vi "Add Transfer Group.vi"(8 "error in (no error)":errorcluster, 9 "Transfer Group":refnum<class "Transfer Group.lvclass">, 10 "parent tag":string, 11 "TreeControl in":refnum<vi>) -> (0 "error out":errorcluster, 2 "new item tag":string, 3 "TreeControl out":refnum<vi>)   [LabVIEW 2021, in "DSF Core.lvlib"]
uses:
  DSF Core.lvlib
  Classes/Transfer Group/Transfer Group.lvclass
  ID to Tree Items/Tree Item Type.ctl
  Classes/Transfer Group/Transfer Group.lvclass/Transfer Group.ctl
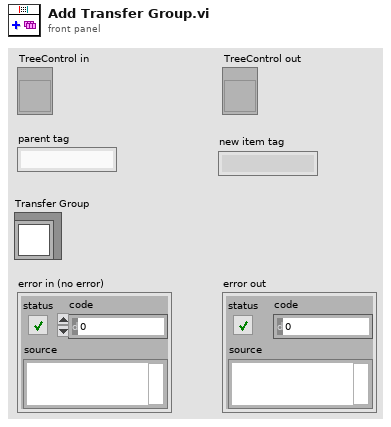
[diagram p1: front panel]
types:
  T1 = typedef "DSF Core.lvlib/Tree Item Type.ctl" = enum16{"Framework", "Plugin Group", "Plugin", "Group", "Transfer", "Buffer", "Channel"}
  T2 = typedef "DSF Core.lvlib/Tree Item.ctl" = cluster{"Left Cell String":string, "Child Text":string[], "Child Tag":string, "Glyph Index":i32}
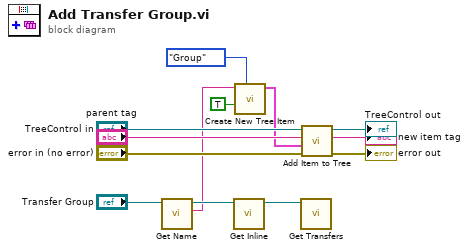
[diagram p0: block diagram]
diagram:
  n1 = call "Get Name.vi"("Transfer Group in"="Transfer Group") -> ("name"=w1:string, "Transfer Group out"=w3:refnum<class "Transfer Group.lvclass">)  [unwired: 9 in]
  n2 = call "Get Inline.vi"("Transfer Group in"=w3) -> ("Transfer Group out"=w2:refnum<class "Transfer Group.lvclass">)  [unwired: 9 in, 1 out]
  n3 = call "Create New Tree Item.vi"("Item Type"=Tree_Item_Type."Group", "found?"=TRUE, "Left Cell String"=w1) -> ("Item"=w7:T2)  [unwired: 7 in, 1 out]
  n4 = call "Get Transfers.vi"("Transfer Group in"=w2) -> ()  [unwired: 9 in, 2 out]
  n5 = call "Add Item to Tree.vi"("error in (no error)"="error in (no error)", "Item"=w7, "parent tag"="parent tag", "TreeControl in"="TreeControl in") -> ("error out"=→"error out":errorcluster, "new item tag"=→"new item tag":string, "TreeControl out"=→"TreeControl out":refnum<vi>)  [unwired: 5 in]
